vi "3.vi"() -> ()   [LabVIEW 2021]
uses:
  1/Control 2.ctl
  1/Control 5.ctl
  Runner's Data.ctl
  HR Data Structure.ctl
  Raw Data.ctl
panel:
  in  "Runner's Data":T1
  out "BPM":cluster{"Time":timestamp[], "Bpm":i32[]}(graph)
  out "XY Graph":T2
  out "error out":errorcluster
  in  "error in (no error)":errorcluster
  out "Heart Rate Zones":T3[][](array[typedef])
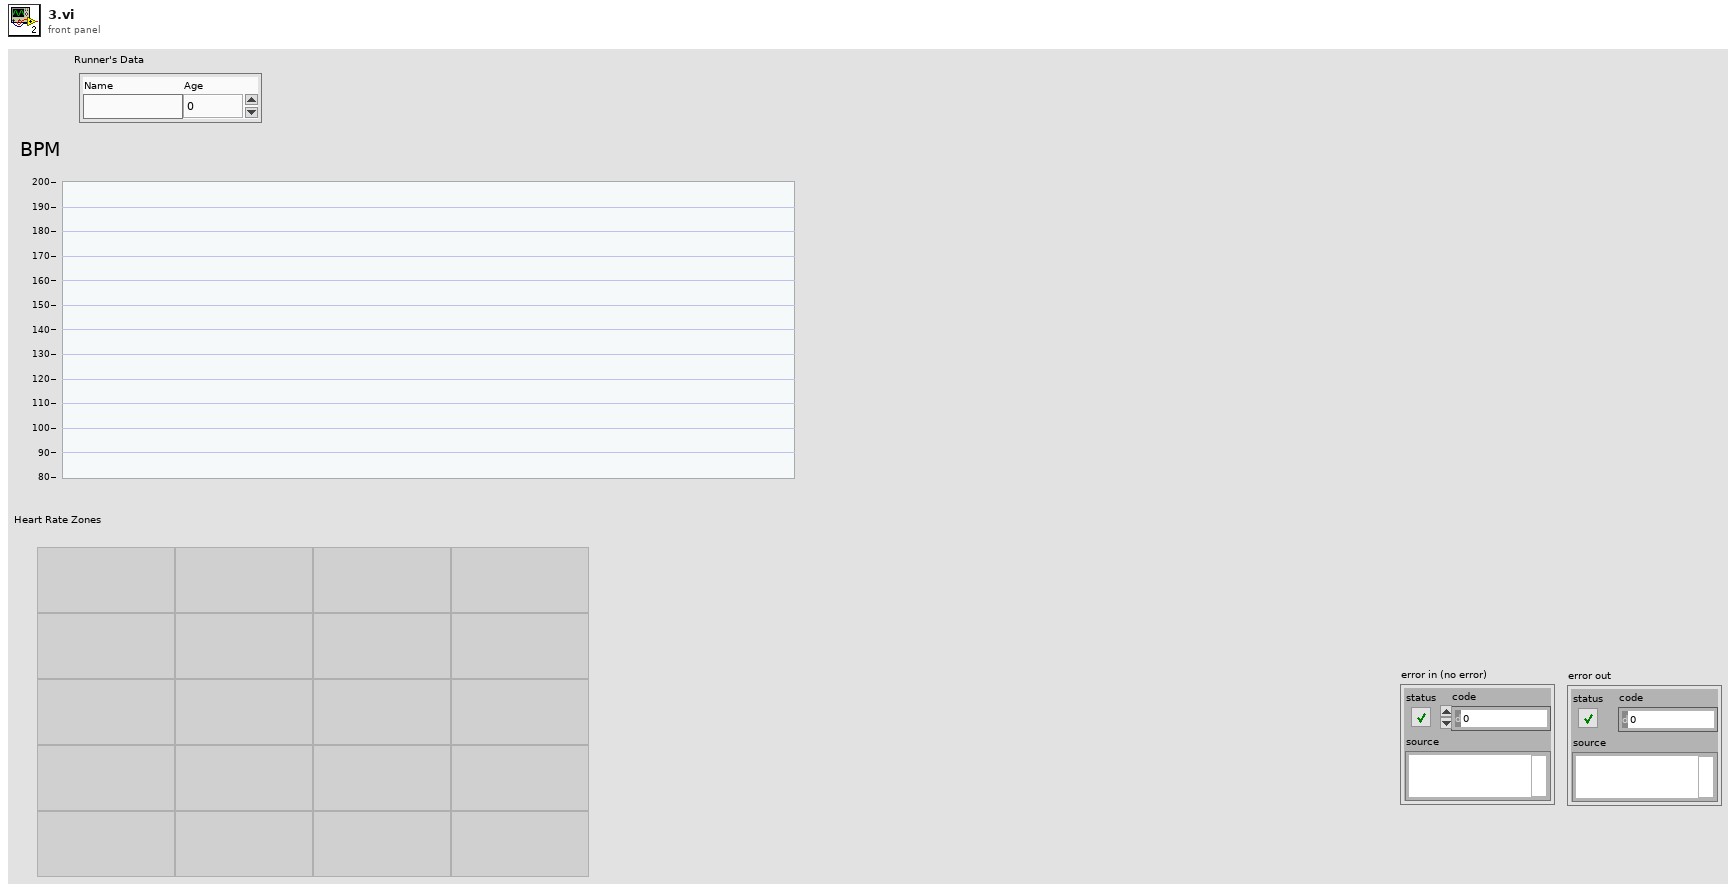
[diagram p1: front panel]
types:
  T1 = typedef "Runner's Data.ctl" = cluster{"Name":string, "Age":i32}
  T2 = typedef "Control 5.ctl" = cluster{"Heart Rate Zone":i32[], " Total time in Zone (%) ":dbl[]}
  T3 = typedef "Control 2.ctl" = string
  T4 = typedef "HR Data Structure.ctl" = cluster{"Runner's Data":T1, "HR Max":i32, "Raw Data":T5, "% HR MAX ":dbl[], "HR Zones Info":string[][], "Heart Rate Zones":dbl[]}
  T5 = typedef "Raw Data.ctl" = cluster{"Time":timestamp[], "Bpm":i32[]}
  T6 = cluster{"Heart Rate Zones No":dbl[], "Raw Data":T5, "HR Zones":string[][]}
  T7 = cluster{"reversed array":dbl[], "Heart Rate Zones No":dbl[]}
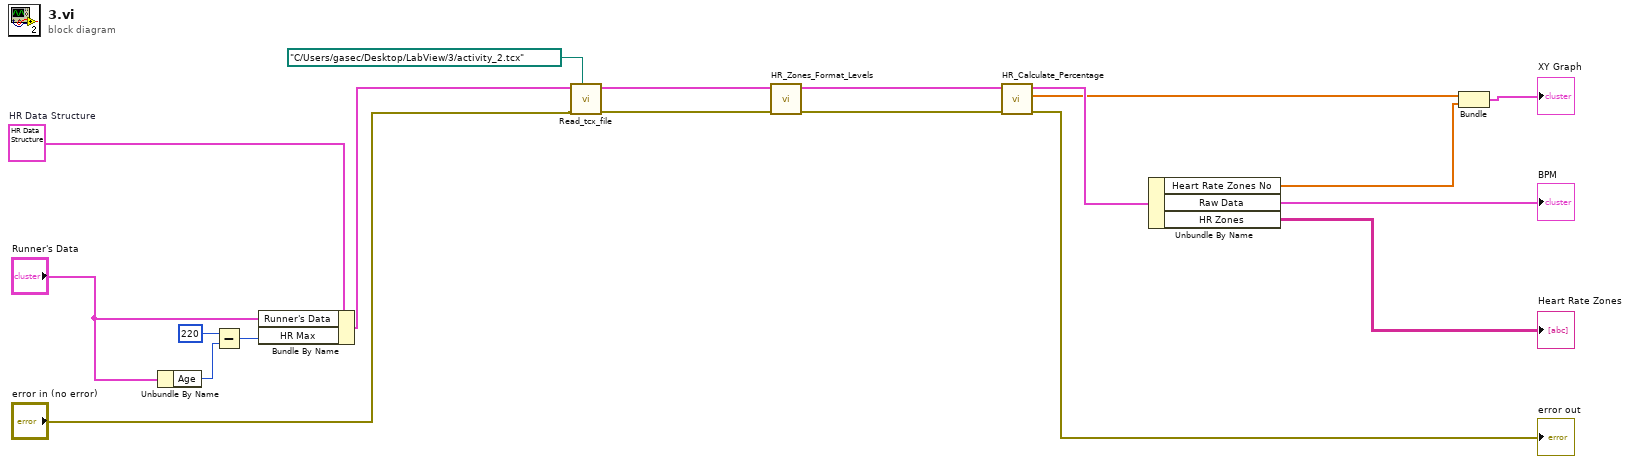
[diagram p0: block diagram]
diagram:
  w1 = T4 data[18170B]  # HR Data Structure
  n1 = Unbundle By Name("Runner's Data") -> ("Age"=w18:i32)
  n2 = Subtract(x=220 ("Age"), y=w18) -> (x-y=w17:i32)
  n3 = Bundle By Name(cluster=w1, "Runner's Data"="Runner's Data", "HR Max"=w17) -> (w5:T4)
  n4 = call "Read_tcx_file.vi"("Path"=path "C:/Users/gasec/Desktop/LabView/3/activity_2.tcx", "error in (no error)"="error in (no error)", "HR Data Structure"=w5) -> ("error out"=w2:errorcluster, "HR Data Structure 2"=w3:T4)  [unwired: 7 in]
  n5 = call "HR_Zones_Format_Levels.vi"("error in (no error)"=w2, "HR Data Structure"=w3) -> ("error out"=w15:errorcluster, "HR Data Structure 2"=w16:T4)  [unwired: 8 in]
  n6 = call "HR_Calculate_Percentage.vi"("error in (no error)"=w15, "HR Data Structure in"=w16) -> ("error out"=→"error out":errorcluster, "reversed array"=w12:dbl[], "output cluster"=w13:T6)  [unwired: 7 in]
  n7 = Unbundle By Name(w13) -> ("Heart Rate Zones No"=w11:dbl[], "Raw Data"=→"BPM":T5, "HR Zones"=→"Heart Rate Zones":string[][])
  n8 = Bundle("reversed array"=w12, "Heart Rate Zones No"=w11) -> (→"XY Graph":T7)  [unwired: 1 in]
